vi "WINDOW-System Config.vi"() -> ()   [LabVIEW 2017]
uses:
  User Interface/Windows/System config window/Typedefs/HW Setup tab control.ctl
  Peripherals Control/Triggers/Typedefs/Triggers output setup.ctl
  Peripherals Control/Triggers/Typedefs/Trigger setup element cluster.ctl
  Typedefs/AOL Properties Cluster.ctl
  Typedefs/CTRL system config cluster.ctl
  Typedefs/DAQ FPGA config cluster.ctl
  <vilib>/userdefined/High Color/nirio_resource_hc.ctl
  Typedefs/FPGA input type AC-DC.ctl
  RIG-SPECIFIC FILES/FPGA Refs/FPGA Ref.ctl
  Peripherals Control/Triggers/Typedefs/General trigger settings cluster.ctl
  Typedefs/Trigger 1 selector enum.ctl
  Typedefs/XY Stage config cluster.ctl
  Typedefs/Z Stage config cluster.ctl
  Typedefs/Laser 1 config cluster.ctl
  Typedefs/PreChirper 1 config cluster.ctl
  Typedefs/Encoder config cluster.ctl
  Typedefs/Laser Power Control HW config.ctl
  Typedefs/Cam VidRec HW config setup cluster.ctl
  Typedefs/Triggers HW config.ctl
  Typedefs/Objective Config.ctl
  Typedefs/AOD Settings-distilled.ctl
  Typedefs/Prechirper Cal Config.ctl
  Typedefs/PreChirper constants.ctl
  Typedefs/CTRL system config.ctl
  Typedefs/Control Sys HW config cluster.ctl
  Typedefs/DAQ FPGA HW config cluster.ctl
  Typedefs/DAQ FPGA system config.ctl
  User Interface/Windows/System config window/Typedefs/HW config window refs cluster.ctl
  User Interface/Visualisation/Functional Imaging Viewer/Typedefs/Get-Set-Clear Control.ctl
  Typedefs/HW config states enum.ctl
  User Interface/Windows/System config window/Globals/Sys Config window globals.vi
  Global Variables/General Globals.vi
  Global Variables/gl_UI Ctrl Refs.vi
panel:
  in  "DAQ FPGA config cluster":T1={"Target"="RIO0", "input card type"=enum."AC Card", "Ref"=refnum, "Clock Freq (MHz) "=200.0, "Samples Wait after Trigger"=5080, "AOD fill"=4900, "StartupDelay"=0, "Slip Cycle (clock cycles)"=600000, "Add Cycle"=TRUE}
  in  "Control system":T5={"Contrl Sys Available Ind"=FALSE, "Control system.FPGA Type"=enum."Virtex 5", "Control system.Network adapter name"="", "Control system.MAC address"="", "Control system.Ethernet Port"=3, "Ethernet opened"=FALSE, "Ctrl FPGA Clock (MHz)"=240.0, "AOD 1 Amplitude"=0, "AOD 2 Amplitude"=0, "AOD 3 Amplitude"=0, "AOD 4 Amplitude"=0, "AOD 5 Amplitude"=0, "AOD 6 Amplitude"=0, "Data Time Interval (ns)"=0.0, "T0 (ns)"=0.0, "Ta (ns)"=0.0} {"Control system.Ethernet Port" min=0 max=2048 step=1; "Ctrl FPGA Clock (MHz)" min=80.0 max=500.0 step=1.0; "Data Time Interval (ns)" min=0.0 max=2048.0 step=1.0; "Ta (ns)" min=0.0 max=2048.0 step=1.0; "T0 (ns)" min=0.0 max=2048.0 step=1.0; "AOD 6 Amplitude" min=0 max=2048 step=1; "AOD 5 Amplitude" min=0 max=2048 step=1; "AOD 4 Amplitude" min=0 max=2048 step=1; "AOD 3 Amplitude" min=0 max=2048 step=1; "AOD 2 Amplitude" min=0 max=2048 step=1; "AOD 1 Amplitude" min=0 max=2048 step=1}
  in  "Cancel":bool
  in  "OK":bool
  in  "AOL Properties":T6={"AOD 1 thickness (mm)"=118.0, "AOD 2 thickness (mm)"=115.0, "AOD 3 thickness (mm)"=110.0, "AOD 4 thickness (mm)"=135.0, "AOD 5 thickness (mm)"=135.0, "AOD 6 thickness (mm)"=135.0, "AOD 1-2 separation (mm)"=15.0, "AOD 2-3 separation (mm)"=15.0, "AOD 3-4 separation (mm)"=15.0, "AOD 4-5 separation (mm)"=15.0, "AOD 5-6 separation (mm)"=15.0, "AOD 1 X Offset"=15.0, "AOD 2 X Offset"=1.0, "AOD 3 X Offset"=1.0, "AOD 4 X Offset"=1.0, "AOD 1 Y Offset"=1.0, "AOD 2 Y Offset"=1.0, "AOD 3 Y Offset"=1.0, "AOD 4 Y Offset"=1.0, "AOD 1 X Direction"=0.0, "AOD 2 X Direction"=0.0, "AOD 3 X Direction"=0.0, "AOD 4 X Direction"=0.0, "AOD 1 Y Direction"=1.0, "AOD 2 Y Direction"=0.0, "AOD 3 Y Direction"=0.0023, "AOD 4 Y Direction"=0.0046, "AOD 1 Centre (mm)"=15.0, "AOD 2 Centre (mm)"=50.0, "AOD 3 Centre (mm)"=50.0, "AOD 4 Centre (mm)"=50.0, "Timing Offset AOD 1"=0.0, "Timing Offset AOD 2"=0.0, "Timing Offset AOD 3"=0.0, "Timing Offset AOD 4"=0.0, "AOD Optical offset 1"=20000.0, "AOD Optical offset 2"=20000.0, "AOL aperture (mm)"=15.0, "AOL centre wavelength (nm)"=1.0, "AOL centre frequency (MHz)"=1.0, "Diffraction mode"=1.0, "Crystal length (mm)"=0.0, "Acoustic velocity (m/s)"=1.0, "Pair deflection ratio"=1.0, "AOD fill time (us)"=1.0, "AOD Ord. Refractive index"=2.22, "AOD ExtraOrd. Refractive index"=2.22}
  in  "Config Tab Control":T7=enum."Hardware Setup"
  in  "Control Sys. HW config":T8
  in  "Controller System Config":T9={"AOD 1 Amplitude"=0, "AOD 2 Amplitude"=0, "AOD 3 Amplitude"=0, "AOD 4 Amplitude"=0, "AOD 5 Amplitude"=0, "AOD 6 Amplitude"=0, "T0 (ns)"=0.0, "Ta (ns)"=0.0, "Data Time Interval (ns)"=0.0, "Ctrl FPGA Clock (MHz)"=240.0} {"Ctrl FPGA Clock (MHz)" min=80.0 max=500.0 step=1.0; "Data Time Interval (ns)" min=0.0 max=2048.0 step=1.0; "Ta (ns)" min=0.0 max=2048.0 step=1.0; "T0 (ns)" min=0.0 max=2048.0 step=1.0; "AOD 6 Amplitude" min=0 max=2048 step=1; "AOD 5 Amplitude" min=0 max=2048 step=1; "AOD 4 Amplitude" min=0 max=2048 step=1; "AOD 3 Amplitude" min=0 max=2048 step=1; "AOD 2 Amplitude" min=0 max=2048 step=1; "AOD 1 Amplitude" min=0 max=2048 step=1}
  in  "Ctrl FPGA available":bool
  in  "DAQ FPGA System Config":T10={"Clock Freq (MHz) "=200.0, "Samples Wait after Trigger"=5080, "AOD fill"=4900, "StartupDelay"=0, "Slip Cycle (clock cycles)"=600000, "Add Cycle"=TRUE}
  in  "DAQ FPGA HW Config":T11={"FGPA Ref"=refnum, "Target"="RIO0", "input card type"=enum."AC Card"}
  in  "Triggers sub-tab control":enum32{"General", "Routing & Timing"}(tab)
  in  "Trigger HW config":T12
  in  "General trigger settings":T13={"Trigger 1 function"=enum."Encoder trigger", "Triggers loop clock (MHz)"=80.0} {"Triggers loop clock (MHz)" format="%#_13g"}
  in  "Triggers output setup":T15 {"Pulse width (us)" min=10 max=5000 step=1 format="%.0fµs"}
  in  "Externalise Triggers":bool
  in  "Galvo AOs":tag
  in  "Power meter AI":tag
  in  "Pockels AO":tag
  in  "PMT AOs":tag
  in  "Hard shutter AO":tag
  in  "Z stage available":bool
  in  "XY stage available":bool
  in  "Z Stage config cluster":T17={"COM port"="COM7", "Baudrate"=0, "Type"=""}
  in  "XY Stage config cluster":T18={"COM port"="COM7", "Baudrate"=0, "Type"=""}
  in  "XY stage COM port":refnum<visa-resource-name>="COM7"
  in  "Encoder":T19={"IP address"="224.0.1.103", "Port"=7000, "Wheel radius (cm)"=16.0, "Encoder Trigger"=""} {"Wheel radius (cm)" format="%#_13g"}
  in  "Wheel radius (cm)":dbl format="%#_13g"
  in  "Encoder IP address":string="224.0.1.103"
  in  "Encoder port":u16=7000
  in  "Encoder available":bool
  in  "Computer MAC address":string="82574L"
  in  "Demo mode":enum16{"Full functionality", "Demo mode"}(ring) caption="Mode"
  in  "Number of AODs":dbl=4.0
  in  "Swap XY on stage":bool
  in  "DO flag-Trial start":tag
  in  "DO flag-Video record":tag
  in  "Cam VidRec available":bool caption="Cameras video recording system is available"
  in  "Cam VidRec":T20
  in  "AOD Settings - distilled":T21={"AOD 1 thickness (mm)"=8.0, "AOD 2 thickness (mm)"=8.0, "AOD 3 thickness (mm)"=8.0, "AOD 4 thickness (mm)"=8.0, "AOD 1-2 separation (mm)"=50.0, "AOD 2-3 separation (mm)"=50.0, "AOD 3-4 separation (mm)"=50.0, "AOD 1 Centre (mm)"=7.5, "AOD 2 Centre (mm)"=7.5, "AOD 3 Centre (mm)"=7.5, "AOD 4 Centre (mm)"=7.5, "AOD 1 X Offset"=0.0, "AOD 2 X Offset"=0.0023, "AOD 3 X Offset"=0.0046, "AOD 4 X Offset"=0.0046, "AOD 1 Y Offset"=0.0, "AOD 2 Y Offset"=0.0, "AOD 3 Y Offset"=0.0023, "AOD 4 Y Offset"=0.0046, "Timing Offset AOD 1"=0.0, "Timing Offset AOD 2"=0.0, "Timing Offset AOD 3"=0.0, "Timing Offset AOD 4"=0.0, "AOL centre wavelength (nm)"=1.0, "AOL centre frequency (MHz)"=1.0, "Pair deflection ratio"=1.0, "AOL aperture (mm)"=15.0, "AOD fill time (us)"=1.0, "Diffraction mode"=1.0, "Crystal length (mm)"=0.0, "Acoustic velocity (m/s)"=1.0, "AOD Ord. Refractive index"=2.22}
  in  "Current Objective":string
  in  "Objective Calibration Settings":T22[](array[typedef])
  in  "Pockels cal.Dwell time (µs)":dbl=0.4 caption="Dwell time (µs)" min=0.05 max=12.0 step=0.1 format="%#.2fµs"
  in  "Pockels cal.Zoom":u8=12 caption="Zoom" min=1 max=24 step=1 format="x%.0f"
  in  "Laser 1 available":bool
  in  "Laser 1 config":T23={"COM port"="COM7", "Baud Rate"=0, "Type"=""}
  in  "Laser Power Control HW config":T24={"Laser Power Control"="Pockels", "Laser Power Modulation Control"=enum."NI"}
  in  "Laser Wavelength 2":u16(ring) caption="Laser Wavelength (nm)" items=["920"]
  in  "Prechirper 1 available":bool
  in  "Prechirper 1 config":T25={"Type"="", "Baud Rate"=0, "COM port"="COM7"}
  in  "PreChirper Preset Calibration Values":T26[](array[typedef])
  in  "Prechirper Constants":T27
  in  "PreChirp Preset Values":bool caption="Use Preset Values"
  in  "Initial Laser Wavelength [nm]":dbl=5.0
  in  "Initial Dwell Time [us]":dbl=5.0
  in  "Error Logging":bool
  in  "Performance Monitoring":bool caption="PC Performance Monitoring"
  in  "Microscope ID":string="003"
  in  "Microscope Type":string="AOLM"
  in  "Revision Number":string="1.0.0.0"
  in  "Advanced Imaging":bool
  in  "Max Allowed Trial Length [s]":dbl=60.0
  in  "Initial Scan Resolution":dbl=512.0
  in  "Initial Acceptance Angle [mrad]":dbl=5.0
  # "This functionality connects the various PXI backplane triggers to physical terminals on the DI/O module.\n\n\nOriginal setup:\nPXI_Trigger 0= Unused\nPXI_Trigger 1= Line trigger\nPXI_Trigger 2= Frame trigger / Cycle trigge\nPXI_Trigger 3= Trial trigger\nPXI_Trigger 4= Start of Experiment trigger\nPXI_Trigger 5= Stimulus trigger"
  # "[HWC]"
  # "[DNT]"
  # "NOTE: The triggers setup is part of the user-profiles functionality.\nSave the current user profile to retain any changes you make above.\nChanges will not be automatically saved."
  # "'Externalise Triggers' must be enabled"
  # "[DNT]"
  # "[HWC]"
  # "[Delete me]"
  # "[Delete me later]"
  # "Thickness (mm)"
  # "X Offset"
  # "Separation (mm)"
  # "Y Offset"
  # "Centre (mm)"
  # "Timing Offset"
  # "Pockels Calibration Conditions"
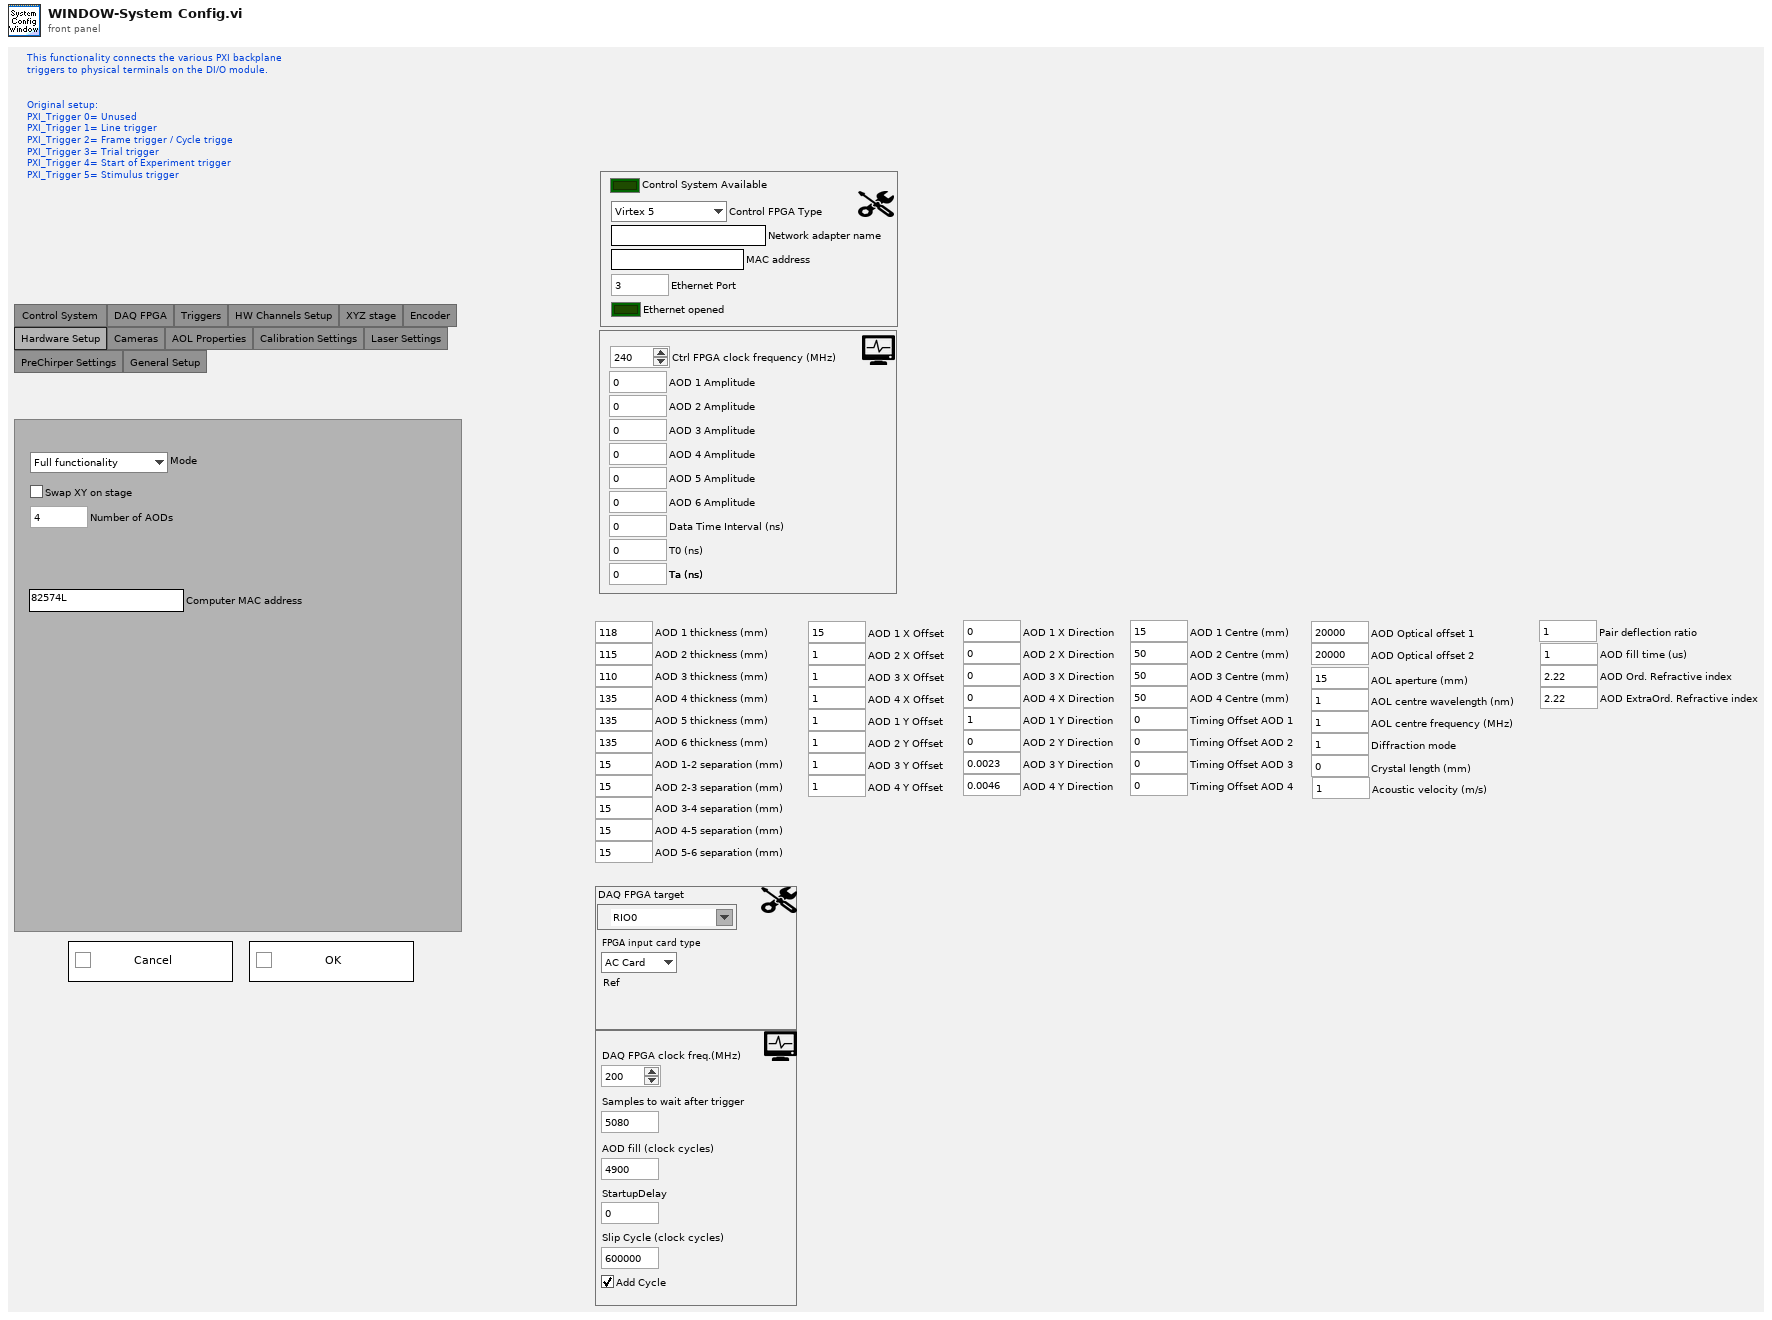
[diagram p1: front panel]
types:
  T1 = typedef "DAQ FPGA config cluster.ctl" = cluster{"Target":T2, "input card type":T3, "Ref":T4, "Clock Freq (MHz) ":dbl, "Samples Wait after Trigger":u16, "AOD fill":u16, "StartupDelay":i32, "Slip Cycle (clock cycles)":u32, "Add Cycle":bool}
  T2 = typedef "nirio_resource_hc.ctl" = tag
  T3 = typedef "FPGA input type AC-DC.ctl" = enum16{"AC Card", "DC Card"}
  T4 = typedef "FPGA Ref.ctl" = refnum<k20>
  T5 = typedef "CTRL system config cluster.ctl" = cluster{"Contrl Sys Available Ind":bool, "Control system.FPGA Type":enum16{"Virtex 5", "Virtex 7"}, "Control system.Network adapter name":string, "Control system.MAC address":string, "Control system.Ethernet Port":i16, "Ethernet opened":bool, "Ctrl FPGA Clock (MHz)":dbl, "AOD 1 Amplitude":i16, "AOD 2 Amplitude":i16, "AOD 3 Amplitude":i16, "AOD 4 Amplitude":i16, "AOD 5 Amplitude":i16, "AOD 6 Amplitude":i16, "Data Time Interval (ns)":dbl, "T0 (ns)":dbl, "Ta (ns)":dbl}
  T6 = typedef "AOL Properties Cluster.ctl" = cluster{"AOD 1 thickness (mm)":dbl, "AOD 2 thickness (mm)":dbl, "AOD 3 thickness (mm)":dbl, "AOD 4 thickness (mm)":dbl, "AOD 5 thickness (mm)":dbl, "AOD 6 thickness (mm)":dbl, "AOD 1-2 separation (mm)":dbl, "AOD 2-3 separation (mm)":dbl, "AOD 3-4 separation (mm)":dbl, "AOD 4-5 separation (mm)":dbl, "AOD 5-6 separation (mm)":dbl, "AOD 1 X Offset":dbl, "AOD 2 X Offset":dbl, "AOD 3 X Offset":dbl, "AOD 4 X Offset":dbl, "AOD 1 Y Offset":dbl, "AOD 2 Y Offset":dbl, "AOD 3 Y Offset":dbl, "AOD 4 Y Offset":dbl, "AOD 1 X Direction":dbl, "AOD 2 X Direction":dbl, "AOD 3 X Direction":dbl, "AOD 4 X Direction":dbl, "AOD 1 Y Direction":dbl, "AOD 2 Y Direction":dbl, "AOD 3 Y Direction":dbl, "AOD 4 Y Direction":dbl, "AOD 1 Centre (mm)":dbl, "AOD 2 Centre (mm)":dbl, "AOD 3 Centre (mm)":dbl, "AOD 4 Centre (mm)":dbl, "Timing Offset AOD 1":dbl, "Timing Offset AOD 2":dbl, "Timing Offset AOD 3":dbl, "Timing Offset AOD 4":dbl, "AOD Optical offset 1":dbl, "AOD Optical offset 2":dbl, "AOL aperture (mm)":dbl, "AOL centre wavelength (nm)":dbl, "AOL centre frequency (MHz)":dbl, "Diffraction mode":dbl, "Crystal length (mm)":dbl, "Acoustic velocity (m/s)":dbl, "Pair deflection ratio":dbl, "AOD fill time (us)":dbl, "AOD Ord. Refractive index":dbl, "AOD ExtraOrd. Refractive index":dbl}
  T7 = typedef "HW Setup tab control.ctl" = enum32{"Control System ", "DAQ FPGA", "Triggers", "HW Channels Setup", "XYZ stage", "Encoder", "Hardware Setup", "Cameras", "AOL Properties", "Calibration Settings", "Laser Settings", "PreChirper Settings", "General Setup"}
  T8 = typedef "Control Sys HW config cluster.ctl" = cluster{"Control system.FPGA Type":enum16{"Virtex 5", "Virtex 7"}, "Control system.Network adapter name":string, "Control system.MAC address":string, "Control system.Ethernet Port":u32, "Control system.Ethernet Port Opened":bool}
  T9 = typedef "CTRL system config.ctl" = cluster{"AOD 1 Amplitude":i16, "AOD 2 Amplitude":i16, "AOD 3 Amplitude":i16, "AOD 4 Amplitude":i16, "AOD 5 Amplitude":i16, "AOD 6 Amplitude":i16, "T0 (ns)":dbl, "Ta (ns)":dbl, "Data Time Interval (ns)":dbl, "Ctrl FPGA Clock (MHz)":dbl}
  T10 = typedef "DAQ FPGA system config.ctl" = cluster{"Clock Freq (MHz) ":dbl, "Samples Wait after Trigger":u16, "AOD fill":u16, "StartupDelay":i32, "Slip Cycle (clock cycles)":u32, "Add Cycle":bool}
  T11 = typedef "DAQ FPGA HW config cluster.ctl" = cluster{"FGPA Ref":T4, "Target":T2, "input card type":T3}
  T12 = typedef "Triggers HW config.ctl" = cluster{"Available Device List":i32, "Device Address":string}
  T13 = typedef "General trigger settings cluster.ctl" = cluster{"Trigger 1 function":T14, "Triggers loop clock (MHz)":dbl}
  T14 = typedef "Trigger 1 selector enum.ctl" = enum16{"Encoder trigger", "Line trigger", "Control system's ref frame acknowledgement"}
  T15 = typedef "Triggers output setup.ctl" = T16[]
  T16 = typedef "Trigger setup element cluster.ctl" = cluster{"Name":string, "Output?":bool, "Output terminal":tag, "PXI backplane line":tag, "Pulse width (us)":u16}
  T17 = typedef "Z Stage config cluster.ctl" = cluster{"COM port":refnum<visa-resource-name>, "Baudrate":i32, "Type":string}
  T18 = typedef "XY Stage config cluster.ctl" = cluster{"COM port":refnum<visa-resource-name>, "Baudrate":i32, "Type":string}
  T19 = typedef "Encoder config cluster.ctl" = cluster{"IP address":string, "Port":u16, "Wheel radius (cm)":dbl, "Encoder Trigger":tag}
  T20 = typedef "Cam VidRec HW config setup cluster.ctl" = cluster{"DO flag-Video record":tag, "DO flag-Trial start":tag}
  T21 = typedef "AOD Settings-distilled.ctl" = cluster{"AOD 1 thickness (mm)":dbl, "AOD 2 thickness (mm)":dbl, "AOD 3 thickness (mm)":dbl, "AOD 4 thickness (mm)":dbl, "AOD 1-2 separation (mm)":dbl, "AOD 2-3 separation (mm)":dbl, "AOD 3-4 separation (mm)":dbl, "AOD 1 Centre (mm)":dbl, "AOD 2 Centre (mm)":dbl, "AOD 3 Centre (mm)":dbl, "AOD 4 Centre (mm)":dbl, "AOD 1 X Offset":dbl, "AOD 2 X Offset":dbl, "AOD 3 X Offset":dbl, "AOD 4 X Offset":dbl, "AOD 1 Y Offset":dbl, "AOD 2 Y Offset":dbl, "AOD 3 Y Offset":dbl, "AOD 4 Y Offset":dbl, "Timing Offset AOD 1":dbl, "Timing Offset AOD 2":dbl, "Timing Offset AOD 3":dbl, "Timing Offset AOD 4":dbl, "AOL centre wavelength (nm)":dbl, "AOL centre frequency (MHz)":dbl, "Pair deflection ratio":dbl, "AOL aperture (mm)":dbl, "AOD fill time (us)":dbl, "Diffraction mode":dbl, "Crystal length (mm)":dbl, "Acoustic velocity (m/s)":dbl, "AOD Ord. Refractive index":dbl}
  T22 = typedef "Objective Config.ctl" = cluster{"Name":string, "Sum X":dbl, "Sum Y":dbl, "Diff X":dbl, "Diff Y":dbl, "Distortion Correction":dbl, "Z_norm to um_scaling":dbl, "X_norm to um_scaling":dbl, "Calibrated Wavelength":dbl}
  T23 = typedef "Laser 1 config cluster.ctl" = cluster{"COM port":refnum<visa-resource-name>, "Baud Rate":i32, "Type":string}
  T24 = typedef "Laser Power Control HW config.ctl" = cluster{"Laser Power Control":string, "Laser Power Modulation Control":enum16{"NI", "FPGA"}}
  T25 = typedef "PreChirper 1 config cluster.ctl" = cluster{"Type":string, "Baud Rate":i32, "COM port":refnum<visa-resource-name>}
  T26 = typedef "Prechirper Cal Config.ctl" = cluster{"Wavelength":i32, "Prism 1":i32, "Prism 2":i32}
  T27 = typedef "PreChirper constants.ctl" = cluster{"a 1":i32, "b 1":i32, "c 1":i32, "a 2":i32, "b 2":i32, "c 2":i32, "lmin":i32, "lmax":i32}
  T28 = typedef "HW config window refs cluster.ctl" = cluster{"VI's reference":refnum<vi>, "menu reference":refnum<k9>, "Pane":refnum<vi>, "Config Tab Control":refnum<vi>, "Triggers sub-tab control":refnum<vi>, "Microscope ID":refnum<vi>, "Microscope Type":refnum<vi>, "Revision Number":refnum<vi>, "Advanced Imaging":refnum<vi>, "Max Allowed Trial Length":refnum<vi>, "Initial Scan Resolution":refnum<vi>, "Initial Acceptance Angle":refnum<vi>, "Initial Laser Wavelength [nm] ":refnum<vi>, "Initial Dwell Time [us]":refnum<vi>, "Error Logging":refnum<vi>, "Performance Monitoring":refnum<vi>, "Ctrl FPGA available":refnum<vi>, "Control HW config":refnum<vi>, "Control System Config":refnum<vi>, "General trigger settings":refnum<vi>, "Trigger HW config":refnum<vi>, "Externalise Triggers":refnum<vi>, "[Triggers output setup]":refnum<vi>, "DAQ FPGA HW Config":refnum<vi>, "DAQ FPGA System Config":refnum<vi>, "Pockels AO":refnum<vi>, "Hard shutter AO":refnum<vi>, "PMT AOs":refnum<vi>, "Galvo AO":refnum<vi>, "Power meter AI":refnum<vi>, "XY stage available":refnum<vi>, "XY Stage config cluster":refnum<vi>, "Z stage available":refnum<vi>, "Z Stage config cluster":refnum<vi>, "Encoder available":refnum<vi>, "Encoder":refnum<vi>, "Encoder IP address":refnum<vi>, "Encoder port":refnum<vi>, "Wheel radius (cm)":refnum<vi>, "Demo mode":refnum<vi>, "Swap XY on stage":refnum<vi>, "Number of AODs":refnum<vi>, "Computer MAC add.":refnum<vi>, "Cam VidRec available":refnum<vi>, "Cam VidRec":refnum<vi>, "DO flag-Video record":refnum<vi>, "DO flag-Trial start":refnum<vi>, "AOD Settings (distilled)":refnum<vi>, "Pockels cal.Dwell time (µs)":refnum<vi>, "Pockels cal.Zoom":refnum<vi>, "Current Objective":refnum<vi>, "[Obj. Calib. Settings]":refnum<vi>, "Laser Wavelength":refnum<vi>, "Laser Power Control \nHW config":refnum<vi>, "Laser 1 available":refnum<vi>, "Laser 1 config":refnum<vi>, "Prechirper 1 available":refnum<vi>, "Prechirper 1 config":refnum<vi>, "PreChirp Preset Values":refnum<vi>, "[PreChirper Preset \nCalibration Values]":refnum<vi>, "Prechirper Constants":refnum<vi>}
  T29 = typedef "Initial config.ctl" = cluster{"Triggers output setup":T15, "General trigger settings":T13, "Calibration settings":T30, "Hardware Configuration":T31, "System Config":T33, "Calibration config.":T34, "General Setup":T35, "AOD Settings - distilled":T21}
  T30 = typedef "Pockels Calibration settings cluster.ctl" = cluster{"Pockels cal.Zoom":u8, "Pockels cal.Dwell time (µs)":dbl}
  T31 = typedef "Hardware Configuration settings.ctl" = cluster{"Dev. PC":bool, "Swap XY on stage":bool, "No of AOD":u8, "Computer MAC address":string, "Externalise Triggers":bool, "Trigger HW config":T12, "DAQmx Chan":T32, "XY stage available":bool, "XY Stage":T18, "Z stage available":bool, "Z Stage config cluster":T17, "Encoder available":bool, "Encoder":T19, "VidRec available":bool, "Cam VidRec":T20, "Laser Power Control HW config":T24, "Laser 1 available":bool, "Laser 1 config cluster":T23, "Prechirper 1 available":bool, "Prechirper 1 config cluster":T25, "Control system.FPGA available?":bool, "Control Sys. HW config":T8, "DAQ FPGA HW Config":T11}
  T32 = typedef "DAQmx physical channels cluster.ctl" = cluster{"Pockels AO":tag, "Hard shutter AO":tag, "PMT AOs":tag, "Galvo AOs":tag, "Power meter AI":tag}
  T33 = typedef "System Configuration.ctl" = cluster{"Laser wavelength (nm)":dbl, "DAQ FPGA System":T10, "Control system":T9}
  T34 = typedef "Calibration config.ctl" = cluster{"Current Objective":string, "Objective Settings":T22[], "PreChirper Values Preset ?":bool, "PreChirper Settings":T26[], "PreChirper Constants":T27}
  T35 = typedef "General Setup.ctl" = cluster{"Microscope ID":string, "Microscope Type":string, "Revision Number":string, "Advanced Imaging":bool, "Error Logging":bool, "Performance Monitoring":bool, "Max Allowed Trial Length":dbl, "Initial Scan Resolution":dbl, "Initial Acceptance Angle":dbl, "Initial Laser Wavelength":dbl, "Initial Dwell Time":dbl}
  T36 = enum32{"Invalid", "Standard", "Closed", "Hidden", "Minimized", "Maximized"}
  T37 = typedef "Get-Set-Clear Control.ctl" = enum16{"Get", "Set", "Clear"}
  T38 = typedef "HW config states enum.ctl" = enum16{"Load from file", "Save to file", "Write all", "Read all", "Write XY stage settings", "Write DAQ FPGA settings", "Write Control FPGA settings", "Write Phys Channels", "Write System Config", "Write HW Config", "Save System Config", "Save HW Config", "Clear", "Compare from file"}
  T39 = typedef "UI ctrl refs cluster.ctl" = cluster{"Top level VI path":path, "Top level VI ref":refnum<vi>, "User menu ref":refnum<k9>, "Sub Panel control":refnum<vi>, "Imaging Param Tab":refnum<vi>, "Occurrence-Start drivers":refnum<k4>, "Occurrence-Speed logging initialised":refnum<k4>, "Occurrence-XYZ stage initialised":refnum<k4>, "Exit button":refnum<vi>, "Status ind":refnum<vi>, "Set as origin":refnum<vi>, "Speed Logging":refnum<vi>, "Time Lapse":refnum<vi>, "Live Imaging":refnum<vi>, "AOL Z Stack":refnum<vi>, "Motor Z Stack":refnum<vi>, "Funct Acq button":refnum<vi>, "Hard Shutter":refnum<vi>, "Virtual Shutter":refnum<vi>, "Laser Power":refnum<vi>, "AOL Mode":refnum<vi>, "Frame Size":refnum<vi>, "Field of View":refnum<vi>, "Dwell Time":refnum<vi>, "Zoom":refnum<vi>, "AOL Z":refnum<vi>, "Objective":refnum<vi>, "Axis":refnum<vi>, "Paths & Names":refnum<vi>, "Experiment folder path (ind.)":refnum<vi>, "Last State (Ind.)":refnum<vi>, "Averages":refnum<vi>, "Angle (degrees)":refnum<vi>, "X centre":refnum<vi>, "Y centre":refnum<vi>, "Plane Mode":refnum<vi>, "# Planes":refnum<vi>, "Z Start":refnum<vi>, "Z Stop":refnum<vi>, "Z Step":refnum<vi>, "PMT 1":refnum<vi>, "PMT 2":refnum<vi>, "Stage XYZ Position":refnum<vi>, "Pockels@Z Start":refnum<vi>, "Pockels@Z Stop":refnum<vi>, "Obtain Z Start":refnum<vi>, "Obtain Z Stop":refnum<vi>, "Live stim.trig.period":refnum<vi>, "Live stim.trig.enable":refnum<vi>, "Funct. Acq. Pockels Modulation":refnum<vi>, "Enable Video Recording":refnum<vi>, "Video Record-Live Imaging":refnum<vi>, "Video Record-Funct acq":refnum<vi>, "AOL Z-stack Chirps Ready (ind)":refnum<vi>, "Center freq ind (nm)":refnum<vi>, "Logging queue (ind)":refnum<vi>, "Back aperture power (ind.)":refnum<vi>, "Power after objective (ind.)":refnum<vi>, "Switch user":refnum<vi>, "Ls1 Conn. Status":refnum<vi>, "Ls1Tuning Status":refnum<vi>, "Ls1 Faults":refnum<vi>, "Ls1 Connection":refnum<vi>, "Ls1 Mode":refnum<vi>, "Ls1 POWER [mW]":refnum<vi>, "Ls1Shutter":refnum<vi>, "Ls1 Wavelength":refnum<vi>, "Ls1 Note":refnum<vi>, "Ls1 Confirm Wav":refnum<vi>, "Ls1 PreChrp Prism1":refnum<vi>, "Ls1 PreChrp Prism2":refnum<vi>, "Ls1 wav top Ind":refnum<vi>, "Ls1 power top Ind":refnum<vi>, "Ls1 Pump peak Hold":refnum<vi>, "Ls1 Status Ind":refnum<vi>, "Ls1 wav cancel":refnum<vi>, "Experiment Type":refnum<vi>, "Biology Information":refnum<vi>}
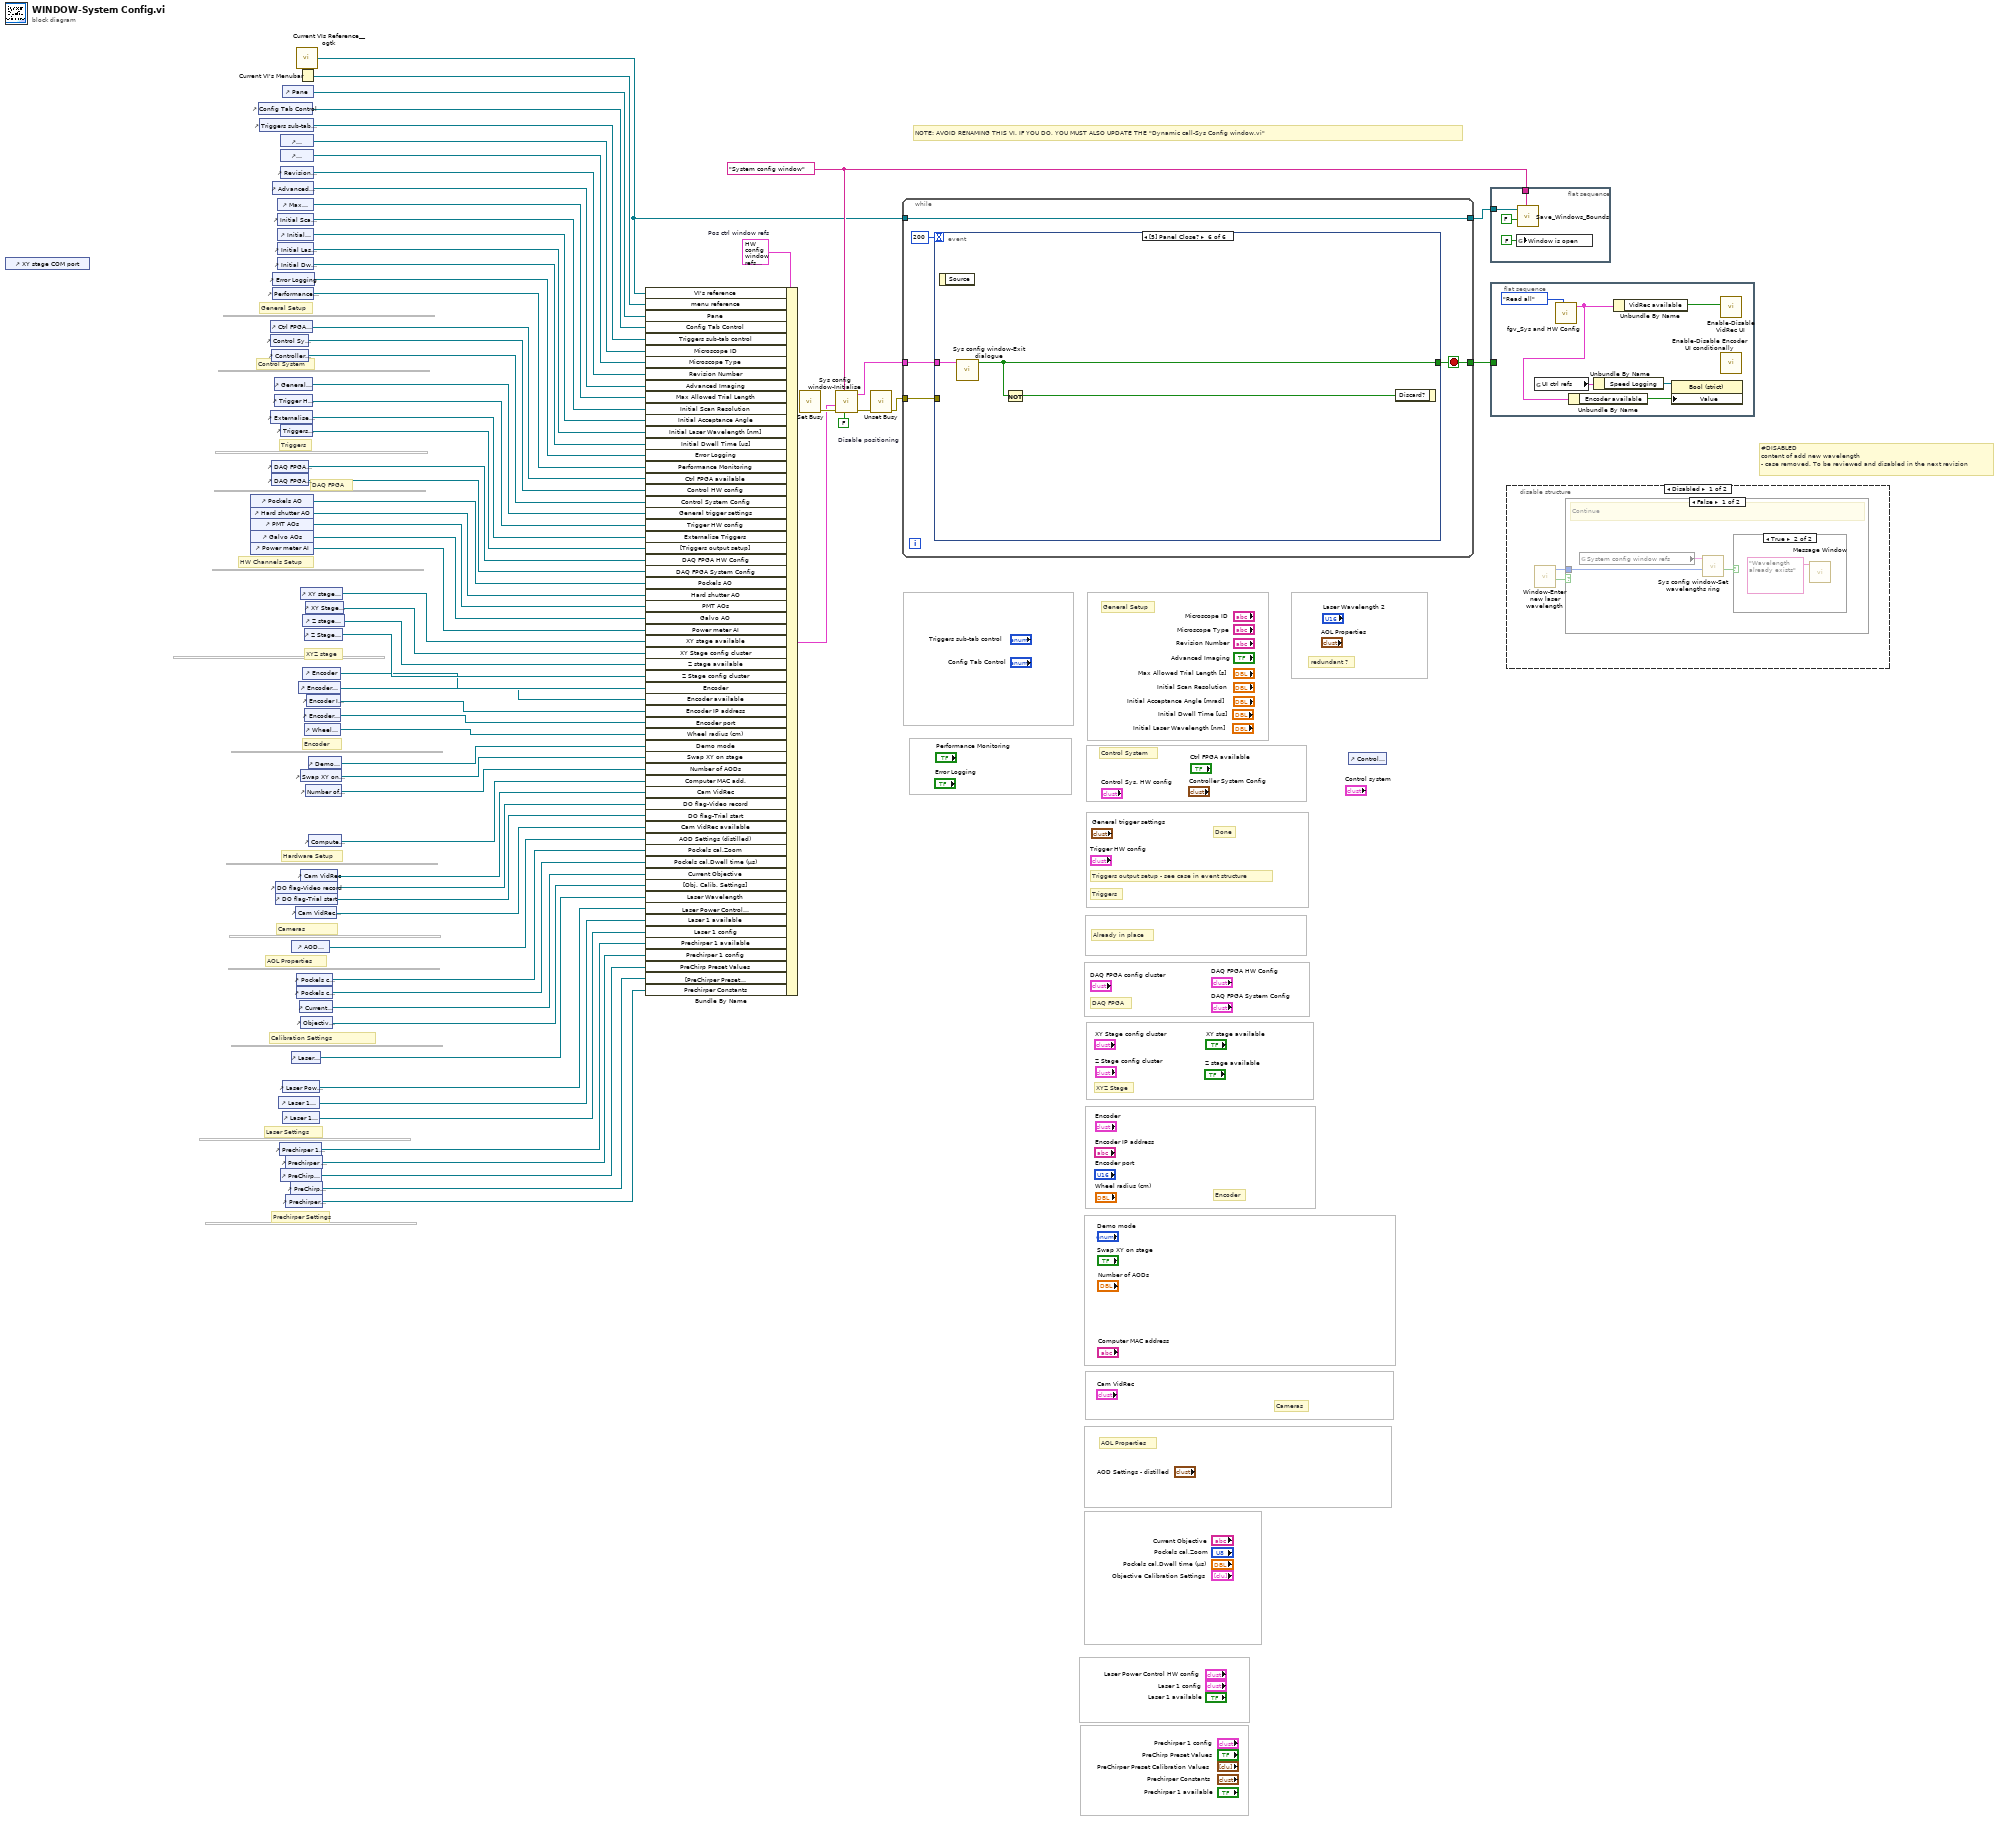
[diagram p0: block diagram]
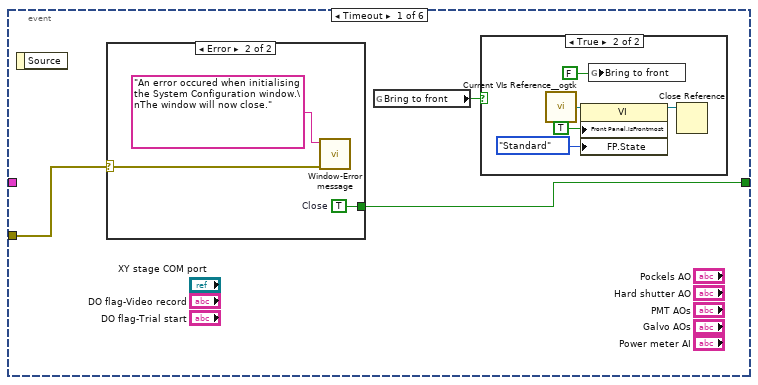
[diagram p5: hidden frame]
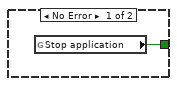
[diagram p7: hidden frame]
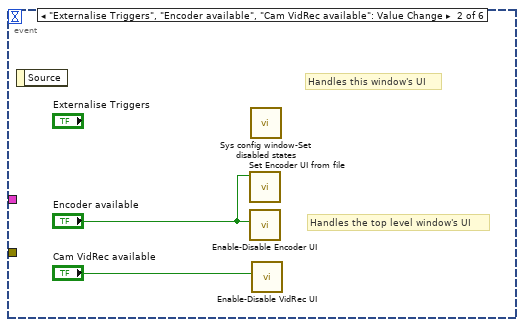
[diagram p8: hidden frame]
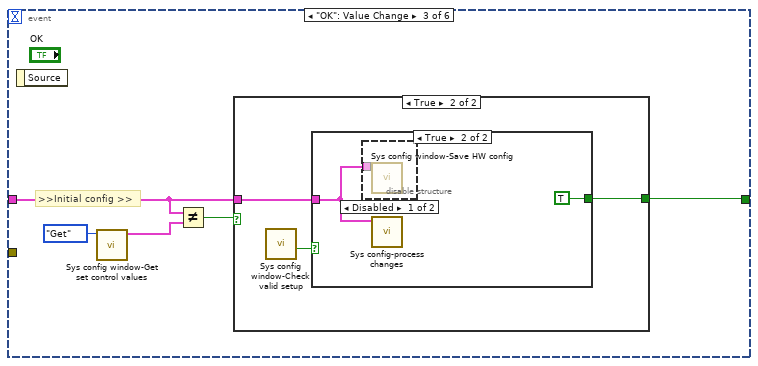
[diagram p9: hidden frame]
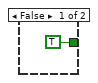
[diagram p10: hidden frame]
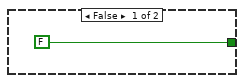
[diagram p11: hidden frame]
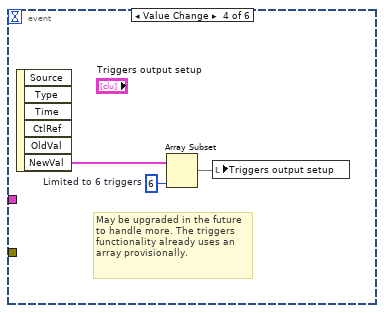
[diagram p13: hidden frame]
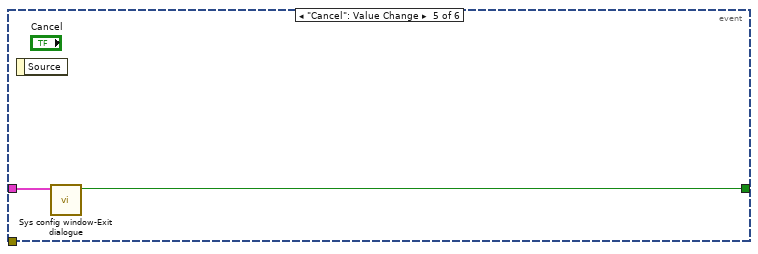
[diagram p14: hidden frame]
diagram:
  w61 = FALSE  # Disable positioning
  w62 = "System config window" ("Window Name (i.e. Key)")
  w71 = T28 {"VI's reference"=refnum, "menu reference"=refnum, "Pane"=refnum, "Config Tab Control"=refnum, "Triggers sub-tab control"=refnum, "Microscope ID"=refnum, "Microscope Type"=refnum, "Revision Number"=refnum, "Advanced Imaging"=refnum, "Max Allowed Trial Length"=refnum, "Initial Scan Resolution"=refnum, "Initial Acceptance Angle"=refnum, "Initial Laser Wavelength [nm] "=refnum, "Initial Dwell Time [us]"=refnum, "Error Logging"=refnum, "Performance Monitoring"=refnum, "Ctrl FPGA available"=refnum, "Control HW config"=refnum, "Control System Config"=refnum, "General trigger settings"=refnum, "Trigger HW config"=refnum, "Externalise Triggers"=refnum, "[Triggers output setup]"=refnum, "DAQ FPGA HW Config"=refnum, "DAQ FPGA System Config"=refnum, "Pockels AO"=refnum, "Hard shutter AO"=refnum, "PMT AOs"=refnum, "Galvo AO"=refnum, "Power meter AI"=refnum, "XY stage available"=refnum, "XY Stage config cluster"=refnum, "Z stage available"=refnum, "Z Stage config cluster"=refnum, "Encoder available"=refnum, "Encoder"=refnum, "Encoder IP address"=refnum, "Encoder port"=refnum, "Wheel radius (cm)"=refnum, "Demo mode"=refnum, "Swap XY on stage"=refnum, "Number of AODs"=refnum, "Computer MAC add."=refnum, "Cam VidRec available"=refnum, "Cam VidRec"=refnum, "DO flag-Video record"=refnum, "DO flag-Trial start"=refnum, "AOD Settings (distilled)"=refnum, "Pockels cal.Dwell time (µs)"=refnum, "Pockels cal.Zoom"=refnum, "Current Objective"=refnum, "[Obj. Calib. Settings]"=refnum, "Laser Wavelength"=refnum, "Laser Power Control \nHW config"=refnum, "Laser 1 available"=refnum, "Laser 1 config"=refnum, "Prechirper 1 available"=refnum, "Prechirper 1 config"=refnum, "PreChirp Preset Values"=refnum, "[PreChirper Preset \nCalibration Values]"=refnum, "Prechirper Constants"=refnum}  # Pos ctrl window refs
  # "#DISABLED\ncontent of add new wavelength\n- case removed. To be reviewed and disabled in the next revision"
  # "Prechirper Settings"
  # "Laser Settings"
  # "Calibration Settings"
  # "AOL Properties"
  # "Cameras"
  # "Hardware Setup"
  # "Encoder"
  # "XYZ stage"
  # "HW Channels Setup"
  # "DAQ FPGA"
  # "Triggers"
  # "Control System"
  # "General Setup"
  # "Done"
  # "redundant ?"
  # "AOL Properties"
  # "Cameras"
  # "Encoder"
  # "Already in place"
  # "XYZ Stage"
  # "DAQ FPGA"
  # "Triggers output setup - see case in event structure"
  # "Triggers"
  # "Control System"
  # "General Setup"
  # "NOTE: AVOID RENAMING THIS VI. IF YOU DO, YOU MUST ALSO UPDATE THE \"Dynamic call-Sys Config window.vi\""
  n1 = control-ref of="XY stage COM port"() -> ()  [unwired: 1 out]
  n2 = control-ref of="Pockels AO"() -> (w45:refnum<vi>)
  n3 = control-ref of="Hard shutter AO"() -> (w44:refnum<vi>)
  n4 = control-ref of="PMT AOs"() -> (w43:refnum<vi>)
  n5 = control-ref of="Galvo AOs"() -> (w42:refnum<vi>)
  n6 = control-ref of="Power meter AI"() -> (w41:refnum<vi>)
  n7 = control-ref of="Config Tab Control"() -> (w14:refnum<vi>)
  n8 = control-ref of="Triggers sub-tab control"() -> (w56:refnum<vi>)
  n9 = control-ref of="Ctrl FPGA available"() -> (w13:refnum<vi>)
  n10 = control-ref of="Control Sys. HW config"() -> (w4:refnum<vi>)
  n11 = control-ref of="Externalise Triggers"() -> (w46:refnum<vi>)
  n12 = control-ref of="Controller System Config"() -> (w3:refnum<vi>)
  n13 = control-ref of="DAQ FPGA HW Config"() -> (w2:refnum<vi>)
  n14 = control-ref of="DAQ FPGA System Config"() -> (w1:refnum<vi>)
  n15 = control-ref of="Advanced Imaging"() -> (w52:refnum<vi>)
  n16 = control-ref of="Performance Monitoring"() -> (w5:refnum<vi>)
  n17 = control-ref of="Error Logging"() -> (w6:refnum<vi>)
  n18 = control-ref of="General trigger settings"() -> (w48:refnum<vi>)
  n19 = control-ref of="Trigger HW config"() -> (w47:refnum<vi>)
  n20 = control-ref of="DO flag-Video record"() -> (w64:refnum<vi>)
  n21 = control-ref of="DO flag-Trial start"() -> (w63:refnum<vi>)
  n22 = control-ref of="Max Allowed Trial Length [s]"() -> (w51:refnum<vi>)
  n23 = control-ref of="Initial Scan Resolution"() -> (w50:refnum<vi>)
  n24 = control-ref of="Initial Acceptance Angle [mrad]"() -> (w49:refnum<vi>)
  n25 = control-ref of="Initial Laser Wavelength [nm]"() -> (w8:refnum<vi>)
  n26 = control-ref of="Initial Dwell Time [us]"() -> (w7:refnum<vi>)
  n27 = control-ref of="Laser 1 available"() -> (w10:refnum<vi>)
  n28 = control-ref of="Prechirper 1 available"() -> (w9:refnum<vi>)
  n29 = control-ref of="Microscope ID"() -> (w55:refnum<vi>)
  n30 = control-ref of="Microscope Type"() -> (w54:refnum<vi>)
  n31 = control-ref of="Revision Number"() -> (w53:refnum<vi>)
  n32 = control-ref of="Triggers output setup"() -> (w22:refnum<vi>)
  n33 = control-ref of="PreChirp Preset Values"() -> (w18:refnum<vi>)
  n34 = control-ref of="Pane"() -> (w65:refnum<vi>)
  n35 = control-ref of="Laser Power Control HW config"() -> (w21:refnum<vi>)
  n36 = control-ref of="Laser 1 config"() -> (w20:refnum<vi>)
  n37 = control-ref of="Prechirper 1 config"() -> (w19:refnum<vi>)
  n38 = control-ref of="Prechirper Constants"() -> (w16:refnum<vi>)
  n39 = control-ref of="PreChirper Preset Calibration Values"() -> (w17:refnum<vi>)
  n40 = control-ref of="Laser Wavelength"() -> (w15:refnum<vi>)
  n41 = control-ref of="AOD Settings - distilled"() -> (w28:refnum<vi>)
  n42 = control-ref of="Cam VidRec available"() -> (w29:refnum<vi>)
  n43 = call <userlib>:"Current VIs Reference__ogtk.vi"() -> ("Current VI's reference"=w60:refnum<vi>)  [unwired: 5 in]
  n44 = control-ref of="Pockels cal.Zoom"() -> (w26:refnum<vi>)
  n45 = control-ref of="Pockels cal.Dwell time (µs)"() -> (w25:refnum<vi>)
  n46 = Current VI's Menubar() -> (w69:refnum<k9>)
  n47 = control-ref of="Encoder available"() -> (w37:refnum<vi>)
  n48 = control-ref of="Current Objective"() -> (w24:refnum<vi>)
  n49 = control-ref of="Swap XY on stage"() -> (w32:refnum<vi>)
  n50 = control-ref of="Cam VidRec"() -> (w30:refnum<vi>)
  n51 = control-ref of="XY stage available"() -> (w12:refnum<vi>)
  n52 = control-ref of="Objective Calibration Settings"() -> (w23:refnum<vi>)
  n53 = control-ref of="Z stage available"() -> (w11:refnum<vi>)
  n54 = control-ref of="Encoder"() -> (w38:refnum<vi>)
  n55 = control-ref of="Encoder port"() -> (w36:refnum<vi>)
  n56 = control-ref of="Wheel radius (cm)"() -> (w34:refnum<vi>)
  n57 = control-ref of="Z Stage config cluster"() -> (w39:refnum<vi>)
  n58 = control-ref of="XY Stage config cluster"() -> (w40:refnum<vi>)
  n59 = control-ref of="Number of AODs"() -> (w31:refnum<vi>)
  n60 = control-ref of="Encoder IP address"() -> (w35:refnum<vi>)
  n61 = control-ref of="Demo mode"() -> (w33:refnum<vi>)
  n62 = control-ref of="Computer MAC address"() -> (w27:refnum<vi>)
  n63 = Bundle By Name(cluster=w71, "VI's reference"=w60, "menu reference"=w69, "Pane"=w65, "Config Tab Control"=w14, "Triggers sub-tab control"=w56, "Microscope ID"=w55, "Microscope Type"=w54, "Revision Number"=w53, "Advanced Imaging"=w52, "Max Allowed Trial Length"=w51, "Initial Scan Resolution"=w50, "Initial Acceptance Angle"=w49, "Initial Laser Wavelength [nm]"=w8, "Initial Dwell Time [us]"=w7, "Error Logging"=w6, "Performance Monitoring"=w5, "Ctrl FPGA available"=w13, "Control HW config"=w4, "Control System Config"=w3, "General trigger settings"=w48, "Trigger HW config"=w47, "Externalise Triggers"=w46, "[Triggers output setup]"=w22, "DAQ FPGA HW Config"=w2, "DAQ FPGA System Config"=w1, "Pockels AO"=w45, "Hard shutter AO"=w44, "PMT AOs"=w43, "Galvo AO"=w42, "Power meter AI"=w41, "XY stage available"=w12, "XY Stage config cluster"=w40, "Z stage available"=w11, "Z Stage config cluster"=w39, "Encoder"=w38, "Encoder available"=w37, "Encoder IP address"=w35, "Encoder port"=w36, "Wheel radius (cm)"=w34, "Demo mode"=w33, "Swap XY on stage"=w32, "Number of AODs"=w31, "Computer MAC add."=w27, "Cam VidRec"=w30, "DO flag-Video record"=w64, "DO flag-Trial start"=w63, "Cam VidRec available"=w29, "AOD Settings (distilled)"=w28, "Pockels cal.Zoom"=w26, "Pockels cal.Dwell time (µs)"=w25, "Current Objective"=w24, "[Obj. Calib. Settings]"=w23, "Laser Wavelength"=w15, "Laser Power Control \nHW config"=w21, "Laser 1 available"=w10, "Laser 1 config"=w20, "Prechirper 1 available"=w9, "Prechirper 1 config"=w19, "PreChirp Preset Values"=w18, "[PreChirper Preset \nCalibration Values]"=w17, "Prechirper Constants"=w16) -> (w57:T28)
  n64 = call <vilib>:"Set Busy.vi"() -> ("error out"=w68:errorcluster)  [unwired: 10 in, 1 out]
  n65 = call "Sys config window-Initialise.vi"("Disable positioning"=w61, "Window Name (i.e. Key)"=w62, "error in (no error)"=w68, "Pos ctrl window refs"=w57) -> ("error out"=w67:errorcluster, "output cluster"=w59:T29)  [unwired: 6 in]
  n66 = call <vilib>:"Unset Busy.vi"("error in (no error)"=w67) -> ("error out"=w66:errorcluster)  [unwired: 10 in]
  n67 = while {
    tunnel: w66 -> [w74]
    tunnel: w60 -> [w76]
    tunnel: [w76] -> w70
    tunnel: w59 -> [w73]
    tunnel: [w72] -> w58
    stop <- w72 stop-if-true
    n68 = event shown="[5] Panel Close?" {
      selector: _ -> [_ _ _ _ _ _]
      dyn-events: _ -> [_ _ _ _ _ _]
      timeout: 200 -> [_ _ _ _ _ _]
      tunnel: [w78 _ w95 _ w108 w109] -> w72
      tunnel: w74 -> [w79 _ _ _ _ _]
      tunnel: w73 -> [_ _ w93 _ w107 w110]
      event Timeout {
        n69 = event-data() -> ()  [unwired: 1 in, 1 out]
        n70 = case shown="Error" w79 {
          selector: w79 -> [_ w87]
          tunnel: [w85 w88] -> w78
          frame No Error {
            n71 = global read "General Globals.vi" "Stop application"() -> (w85:bool)
          }
          frame Error {
            w88 = TRUE  # Close
            n72 = call "Window-Error message.vi"("error in (no error)"=w87, "Message"="An error occured when initialising the System Configuration window.\nThe window will now close." ("Error Source")) -> ()  [unwired: 9 in, 1 out]
          }
        }
        n73 = global read "Sys Config window globals.vi" "Bring to front"() -> (w77:bool)
        n74 = case shown="True" w77 {
          frame False {
          }
          frame True {
            n75 = call <userlib>:"Current VIs Reference__ogtk.vi"() -> ("Current VI's reference"=w84:refnum<vi>)  [unwired: 5 in]
            n76 = property class="VI"(reference=w84, "Front Panel.IsFrontmost"=TRUE ("Front Panel Window:Is Frontmost"), "FP.State"=T36."Standard" ("Front Panel Window:State")) -> (reference out=w83:refnum<vi>)  [unwired: 1 in, 1 out]
            n77 = global write "Sys Config window globals.vi" "Bring to front"(FALSE ("Bring to front")) -> ()
            n78 = Close Reference(reference=w83) -> ()  [unwired: 1 in, 1 out]
          }
        }
      }
      event "Externalise Triggers", "Encoder available", "Cam VidRec available": Value Change {
        # "Handles the top level window's UI"
        # "Handles this window's UI"
        n79 = event-data() -> ()  [unwired: 1 in, 1 out]
        n80 = call "Set Encoder UI from file.vi"("Encoder available"="Encoder available") -> ()  [unwired: 10 in, 1 out]
        n81 = call "Enable-Disable Encoder UI.vi"("Cam VidRec.VidRec available"="Encoder available") -> ()  [unwired: 10 in, 1 out]
        n82 = call "Sys config window-Set disabled states.vi"() -> ()  [unwired: 11 in, 1 out]
        n83 = call "Enable-Disable VidRec UI.vi"("Cam VidRec.VidRec available"="Cam VidRec available") -> ()  [unwired: 11 in]
      }
      event "OK": Value Change {
        # ">>Initial config >>"
        n84 = event-data() -> ()  [unwired: 1 in, 1 out]
        n85 = call "Sys config window-Get set control values.vi"("Function"=Get-Set-Clear_Control."Get") -> ("output cluster"=w92:T29)  [unwired: 9 in, 1 out]
        n86 = Not Equal?(x=w93, y=w92) -> (x != y?=w91:bool)
        n87 = case shown="True" w91 {
          tunnel: [TRUE w98] -> w95
          tunnel: w93 -> [_ w97]
          frame False {
          }
          frame True {
            n88 = call "Sys config window-Check valid setup.vi"() -> ("Continue"=w99:bool)  [unwired: 11 in]
            n89 = case shown="True" w99 {
              tunnel: [FALSE TRUE] -> w98
              tunnel: w97 -> [_ w101]
              frame False {
              }
              frame True {
                n90 = disable-structure shown="Disabled" {
                  disable-tunnel: w101 -> [w103 _]
                  frame Disabled {
                    n91 = call "Sys config window-Save HW config.vi"("Initial Configuration"=w103) -> ()  [unwired: 11 in]
                  }
                  frame Enabled {
                  }
                }
                n92 = call "Sys config-process changes.vi"("Initial Configuration"=w101) -> ()  [unwired: 11 in]
              }
            }
          }
        }
      }
      event Value Change {
        w105 = 6  # Limited to 6 triggers
        # "May be upgraded in the future to handle more. The triggers functionality already uses an array provisionally."
        n93 = event-data() -> ("NewVal"=w106:T15)  [unwired: 1 in, 5 out]
        n94 = Array Subset(array=w106, length=w105) -> (w104:T15)  [unwired: 1 in]
        n95 = local write "Triggers output setup"(w104) -> ()
      }
      event "Cancel": Value Change {
        n96 = event-data() -> ()  [unwired: 1 in, 1 out]
        n97 = call "Sys config window-Exit dialogue.vi"("Initial Configuration"=w107) -> ("Close"=w108:bool)  [unwired: 10 in]
      }
      event Panel Close? {
        n98 = event-data() -> ()  [unwired: 1 in, 1 out]
        n99 = call "Sys config window-Exit dialogue.vi"("Initial Configuration"=w110) -> ("Close"=w109:bool)  [unwired: 10 in]
        n100 = Not(x=w109) -> (.not. x?=w111:bool)
        n101 = event-data("Discard?"=w111) -> ()  [unwired: 1 in, 1 out]
      }
    }
  }
  n102 = control-ref of="Control system"() -> ()  [unwired: 1 out]
  n103 = flat-sequence {
    tunnel: w70 -> [w115]
    tunnel: w62 -> [w113]
    frame #0 {
      n104 = global write "Sys Config window globals.vi" "Window is open"(FALSE ("Bring to front")) -> ()
      n105 = call "Save_Windows_Bounds.vi"("Window Name (i.e. Key)"=w113, "Front Panel Window:Open"=FALSE, "Window VI's Ref"=w115) -> ()  [unwired: 8 in, 1 out]
    }
  }
  n106 = flat-sequence {
    tunnel: w58 -> [_]
    frame #0 {
      n107 = global read "gl_UI Ctrl Refs.vi" "UI ctrl refs"() -> (w118:T39)
      n108 = call "fgv_Sys and HW Config.vi"("Function"=HW_config_states_enum."Read all") -> ("Hardware Configuration OUT"=w116:T31)  [unwired: 8 in, 2 out]
      n109 = Unbundle By Name(w116) -> ("Encoder available"=w117:bool)
      n110 = Unbundle By Name(w118) -> ("Speed Logging"=w119:refnum<vi>)
      n111 = Unbundle By Name(w116) -> ("VidRec available"=w121:bool)
      n112 = property class="Bool (strict)"(reference=w119, "Value"=w117) -> ()  [unwired: 1 in, 2 out]
      n113 = call "Enable-Disable VidRec UI.vi"("Cam VidRec.VidRec available"=w121) -> ()  [unwired: 11 in]
      n114 = call "Enable-Disable Encoder UI conditionally.vi"() -> ()  [unwired: 11 in, 1 out]
    }
  }
  n115 = disable-structure shown="Disabled" {
    frame Disabled {
      n116 = call "Window-Enter new laser wavelength.vi"() -> ("Cancelled"=w122:bool, "Laser wavelength (nm)"=w123:u16)  [unwired: 9 in, 1 out]
      n117 = case shown="False" w122 {
        tunnel: w123 -> [w125 _]
        frame False {
          # "Continue"
          n118 = global read "Sys Config window globals.vi" "System config window refs"() -> (w126:T28)
          n119 = call "Sys config window-Set wavelengths ring.vi"("Laser wavelength (nm)"=w125, "System Config window refs"=w126) -> ("Wavelength already exists"=w124:bool)  [unwired: 9 in]
          n120 = case shown="True" w124 {
            frame False {
            }
            frame True {
              n121 = call "Message Window.vi"("Message string"="Wavelength already exists") -> ()  [unwired: 10 in, 1 out]
            }
          }
        }
        frame True {
          # "Cancelled"
        }
      }
    }
    frame Enabled {
    }
  }
